vi "Read Slave ID.vi"(8 "error in (no error)":errorcluster, 11 "MB_TCP_Master in":refnum<class "MB_Master_TCP.lvclass">) -> (0 "error out":errorcluster, 2 "Slave ID":u8=1, 3 "MB_TCP_Master out":refnum<class "MB_Master_TCP.lvclass">)   [LabVIEW 2023, in "Jiaxin_Stepper_Controller.lvlib" / "MB Master.lvlib" / "MB_Master_TCP.lvclass"]
uses:
  MB_Master_TCP.lvclass
  MB_Master_TCP.lvclass/MB_Master_TCP.ctl
  MB_ADU/MB_ADU.lvclass/MB_ADU.ctl
  MB_ADU_TCP/MB_ADU_TCP.lvclass
  C:/Users/quantum/Documents/SinglePhotonUI/Plasmionique/MB Master/MB_ADU/MB_ADU.lvclass
  MB_ADU/MB_ADU.lvclass
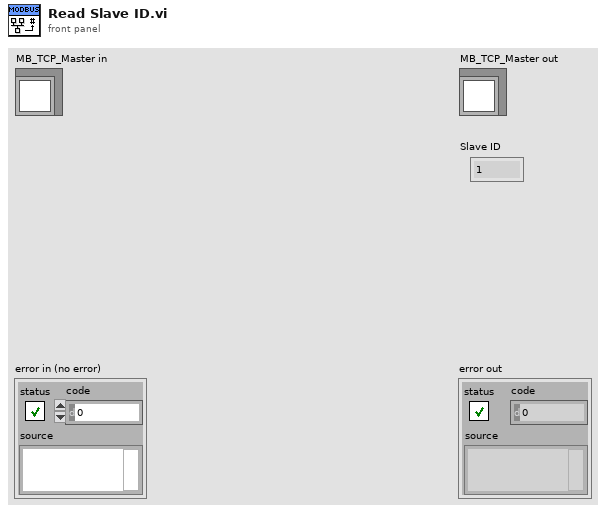
[diagram p1: front panel]
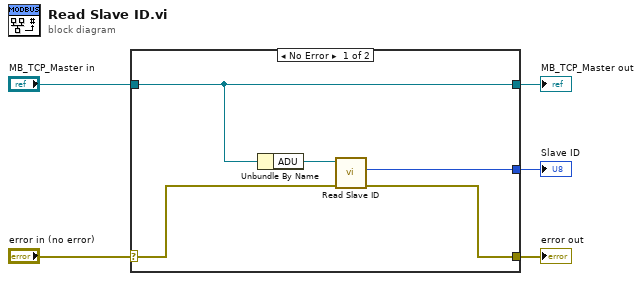
[diagram p0: block diagram]
diagram:
  n1 = case shown="No Error" "error in (no error)" {
    selector: "error in (no error)" -> [w9 w11]
    tunnel: [w8 w11] -> w4
    tunnel: [w6 w12] -> w2
    tunnel: "MB_TCP_Master in" -> [w6 w12]
    tunnel: [w7 _] -> w1
    frame No Error {
      n2 = Unbundle By Name(w6) -> ("ADU"=w10:refnum<class "MB_ADU_TCP.lvclass">)
      n3 = call "Read Slave ID.vi"("error in (no error)"=w9, "MB_ADU_Serial in"=w10) -> ("error out"=w8:errorcluster, "Slave Address"=w7:u8)  [unwired: 7 in, 1 out]
    }
    frame Error {
    }
  }
  "error out" <- w4
  "MB_TCP_Master out" <- w2
  "Slave ID" <- w1
